vi "Execute.vi"(8 "error in":errorcluster, 11 "Set Rel QO2 flow in":refnum<class "Set Rel QO2 flow.lvclass">) -> (0 "error out":errorcluster, 1 "Next Step?":bool, 2 "MSG":string, 3 "Set Rel QO2 flow out":refnum<class "Set Rel QO2 flow.lvclass">)   [LabVIEW 2015, in "Set Rel QO2 flow.lvclass"]
uses:
  Set Rel QO2 flow.lvclass
  Controls/MFC Address.ctl
  Reusable/Sequence/STEPS/LEAVES/Double/Switch DBL.lvclass/Switch DBL.ctl
  Set Rel QO2 flow.lvclass/Set Rel QO2 flow.ctl
  Reusable/Sequence/STEPS/LEAVES/Double/Read val.vi
  Read QO2 DVR.vi
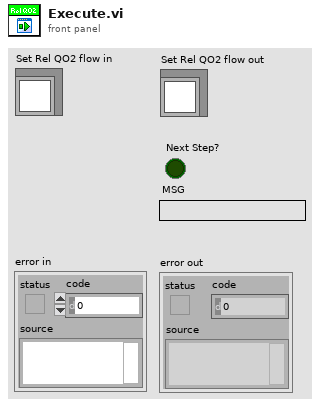
[diagram p1: front panel]
types:
  T1 = typedef "MFC Address.ctl" = enum16{"CRDS Purge", "CRDS Thermodenuded", "CRDS Dry", "CRDS Med RH", "CRDS High RH", "PAS Ch 1", "PAS Ch 2", "PAS Ch3", "PAS Ch 4", "PAS Ch 5", "CLAP", "O3", "Pinlet"}
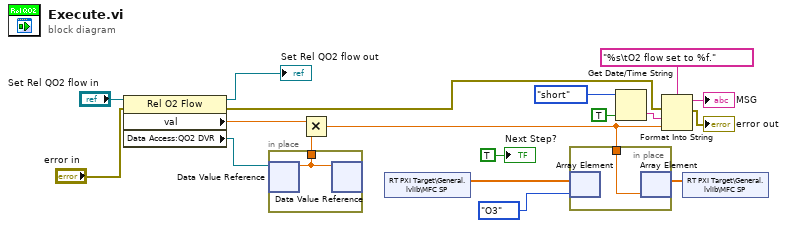
[diagram p0: block diagram]
diagram:
  n1 = property class="Rel O2 Flow"(reference="Set Rel QO2 flow in", error in="error in") -> (reference out=→"Set Rel QO2 flow out":refnum<class "Set Rel QO2 flow.lvclass">, error out=w7:errorcluster, "val"=w13:dbl, "Data Access:QO2 DVR"=w15:refnum<data-value>)
  n2 = in-place {
    in-place-border: [w19] -> w14
    n3 = in-place-dvr #1(w15) -> (w19:dbl)  [unwired: 1 out]
    n4 = in-place-dvr #1(w19) -> ()  [unwired: 2 out]
  }
  n5 = Multiply(x=w13, y=w14) -> (x*y=w3:dbl)
  n6 = shared-variable "RT PXI Target\\General.lvlib\\MFC SP"() -> (w4:sgl[])  [unwired: 1 in, 1 out]
  n7 = in-place {
    in-place-border: w3 -> [w20]
    n8 = in-place-array #2(w4, MFC_Address."O3" ("Controllers")) -> ()  [unwired: 1 out]
    n9 = in-place-array #2(w20) -> (w2:sgl[])  [unwired: 1 out]
  }
  n10 = Get Date/Time String(date format (0)=enum16{"short", "long", "abbreviated"}."short", want seconds? (F)=TRUE) -> (time string=w9:string)  [unwired: 1 in, 1 out]
  n11 = Format Into String(format string="%s\tO2 flow set to %f.", error in=w7, w9, w3) -> (resulting string=→"MSG":string, error out=→"error out":errorcluster)  [unwired: 1 in]
  n12 = shared-variable "RT PXI Target\\General.lvlib\\MFC SP"(w2) -> ()  [unwired: 1 in, 1 out]
  "Next Step?" <- TRUE ("Next Step?")
